vi "Initialise.vi"(8 "error in (no error)":errorcluster, 10 "Instrument Ref":string, 11 "APS7050 in":refnum<class "APS7050.lvclass">) -> (0 "error out":errorcluster, 3 "APS7050 out":refnum<class "APS7050.lvclass">)   [LabVIEW 2019, in "Concrete.lvlib" / "APS7050.lvclass"]
uses:
  APS7050.lvclass
  APS7050.lvclass/APS7050.ctl
  Harware Abstraction/Analog out/Analog out.lvclass
  <instrlib>/APS-7000 Series/APS-7000 Series.lvlib
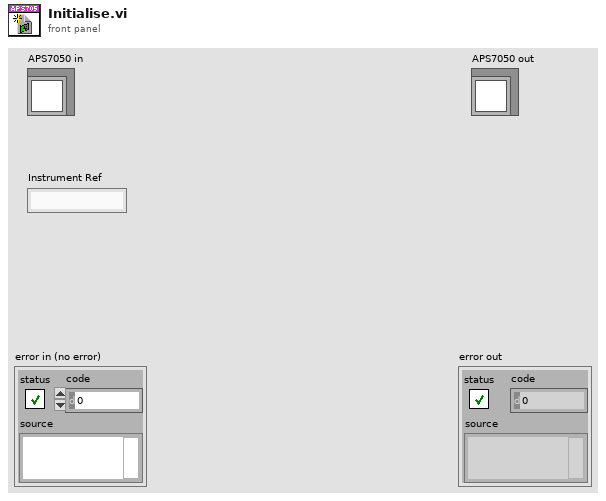
[diagram p1: front panel]
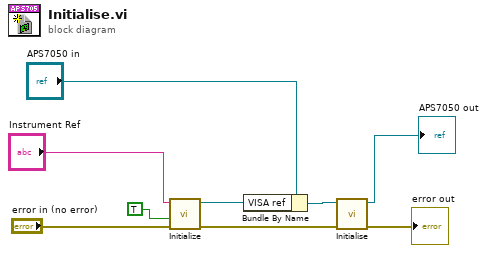
[diagram p0: block diagram]
diagram:
  n1 = call <instrlib>:"Initialize.vi"("error in (no error)"="error in (no error)", "Reset (True)"=TRUE ("ID Query (True)"), "VISA resource name"="Instrument Ref") -> ("error out"=w2:errorcluster, "VISA resource name out"=w4:refnum<visa-resource-name>)  [unwired: 7 in]
  n2 = Bundle By Name(cluster="APS7050 in", "VISA ref"=w4) -> (w8:refnum<class "APS7050.lvclass">)
  n3 = call-parent "Initialise.vi"("error in (no error)"=w2, "Instrument in"=w8) -> ("error out"=→"error out":errorcluster, "Instrument out"=→"APS7050 out":refnum<class "APS7050.lvclass">)  [unwired: 8 in]
